vi "Compile Communication Configuration.vi"(8 "error in (no error)":errorcluster, 11 "Device Ref in":T1 format="%.0x") -> (0 "error out":errorcluster, 2 "Communication Configuration":T2, 3 "Device Ref out":T1 format="%.0x")   [LabVIEW 2019, in "SLSC Switch System Explorer.lvlib"]
uses:
  SLSC Switch System Explorer.lvlib
  Shared/Communication Configuration.ctl
  <vilib>/NI VeriStand/Custom Device API/Custom Device Item Ref.ctl
  Shared/SLSC Switch Shared.lvlib
  <vilib>/NI VeriStand/Custom Device API/Custom Device API.lvlib
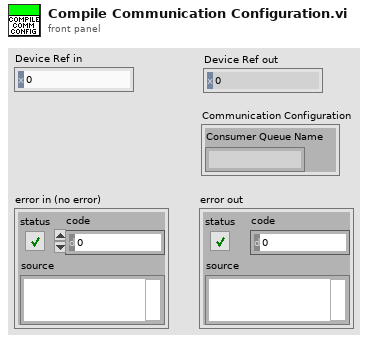
[diagram p1: front panel]
types:
  T1 = typedef "Custom Device API.lvlib/Custom Device Item Ref.ctl" = u64
  T2 = typedef "SLSC Switch Shared.lvlib/Communication Configuration.ctl" = cluster{"Consumer Queue Name":string}
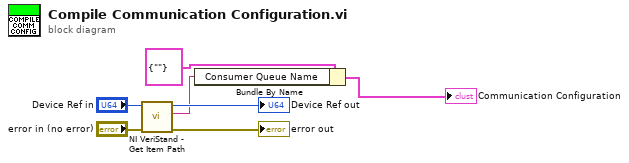
[diagram p0: block diagram]
diagram:
  n1 = call <vilib>:"NI VeriStand - Get Item Path.vi"("error in (no error)"="error in (no error)", "Item Ref in"="Device Ref in") -> ("error out"=→"error out":errorcluster, "Path"=w2:string, "Item Ref out"=→"Device Ref out":T1)  [unwired: 6 in, 1 out]
  n2 = Bundle By Name(cluster=T2 {"Consumer Queue Name"=""} ("Communication Configuration"), "Consumer Queue Name"=w2) -> (→"Communication Configuration":T2)
